vi "get_data.vi"(11 "JSON":variant) -> (0 "Standards [%]":map{string, i32}(c390), 1 "Indexes":map{string, variant}(c390), 3 "Conditions":map{string, i32}(c390), 5 "Timestamps":map{string, string}(c390))   [LabVIEW 2019]
uses:
  <vilib>/LVH/i3 JSON/JSON Parsing/Get Object Parameter Files/Get Object Parameter - Array.vi
  <vilib>/LVH/i3 JSON/JSON Parsing/Get Array Value at Index Files/Get Array Value at Index - Object.vi
  <vilib>/LVH/i3 JSON/JSON Parsing/Get Object Parameter Files/Get Object Parameter - Numeric.vi
  <vilib>/LVH/i3 JSON/JSON Parsing/Get Object Parameter Files/Get Object Parameter - String.vi
  <vilib>/LVH/i3 JSON/JSON Parsing/Get Object Parameter Files/Get Object Parameter - Object.vi
  <vilib>/LVH/i3 JSON/i3-json.lvlib
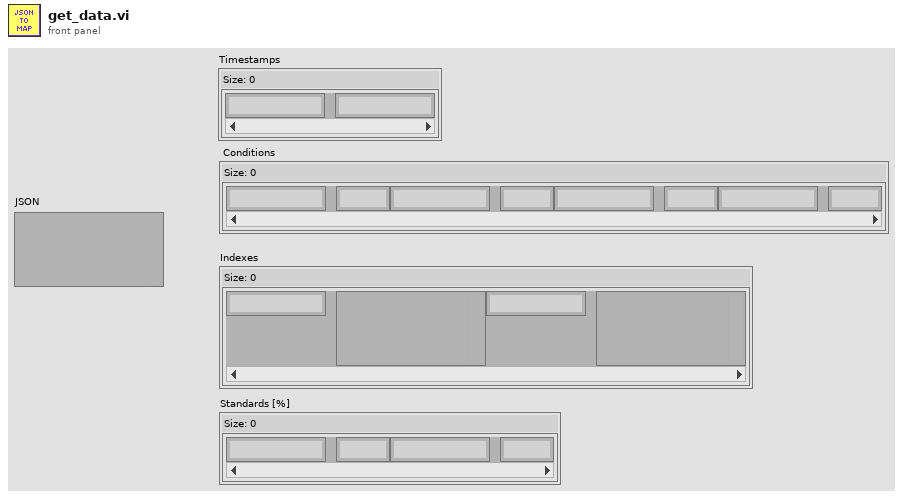
[diagram p1: front panel]
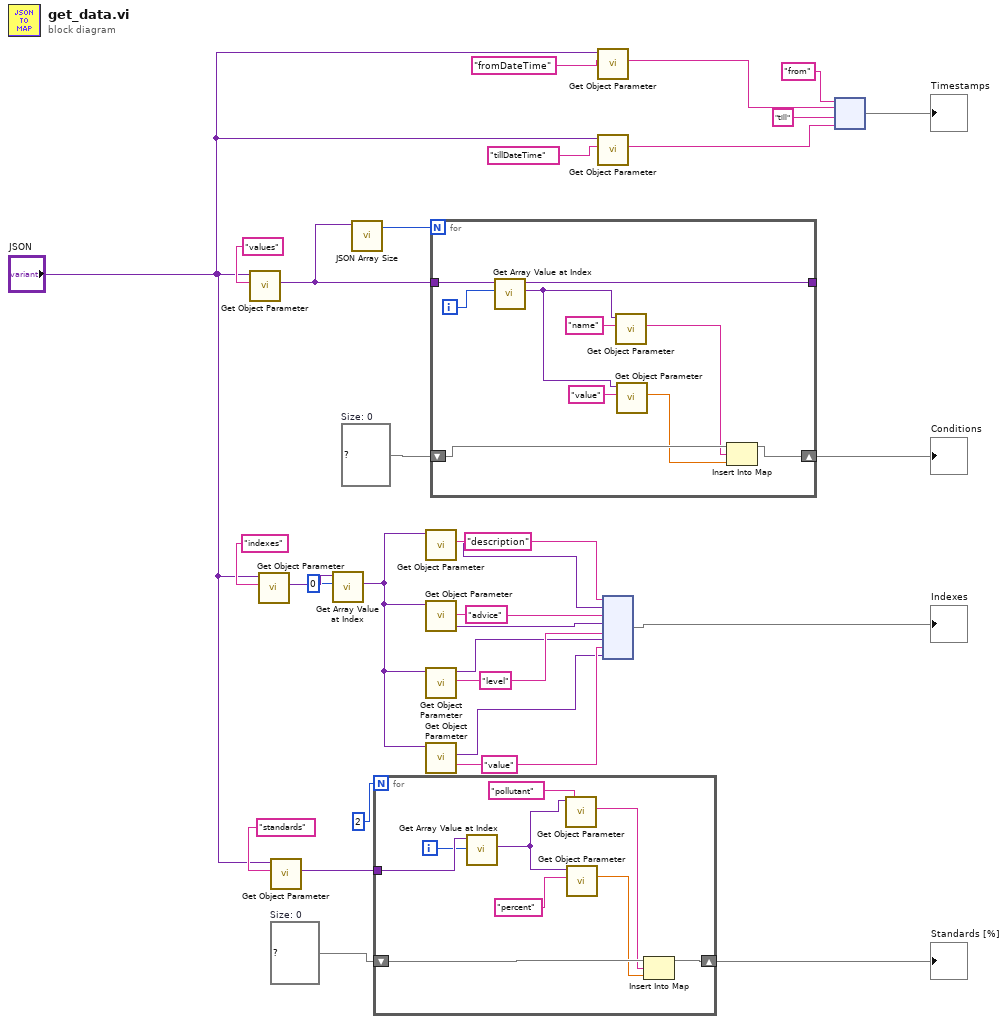
[diagram p0: block diagram]
diagram:
  w10 = map{string, i32} {}  # Size: 0
  w15 = "value" ("Parameter Name")
  w18 = "level" ("Parameter Name")
  w20 = "advice" ("Parameter Name")
  w22 = "description" ("Parameter Name")
  w28 = map{string, i32} {}  # Size: 0
  n1 = call-poly <vilib>:"Get Object Parameter.vi"("Parameter Name"="values", "JSON Tree In (JSON Object)"="JSON") -> ("JSON Array"=w29:variant)  [unwired: 6 in, 3 out]
  n2 = call-poly <vilib>:"Get Object Parameter.vi"("Parameter Name"="indexes", "JSON Tree In (JSON Object)"="JSON") -> ("JSON Array"=w26:variant)  [unwired: 6 in, 3 out]
  n3 = call-poly <vilib>:"Get Object Parameter.vi"("Parameter Name"="standards", "JSON Tree In (JSON Object)"="JSON") -> ("JSON Array"=w12:variant)  [unwired: 6 in, 3 out]
  n4 = call-poly <vilib>:"Get Array Value at Index.vi"("Index"=0, "JSON Tree In (JSON Array)"=w26) -> ("JSON Object"=w23:variant)  [unwired: 6 in, 3 out]
  n5 = call <vilib>:"JSON Array Size.vi"("JSON Tree In (JSON Array)"=w29) -> ("Array Size"=w30:i32)  [unwired: 8 in, 2 out]
  n6 = for {
    N: 2 -> [_]
    tunnel: w12 -> [w40]
    shift-right: [w37] -> w9
    shift-left: w10 -> [w38]
    i -> [w39]
    n7 = call-poly <vilib>:"Get Array Value at Index.vi"("Index"=w39, "JSON Tree In (JSON Array)"=w40) -> ("JSON Object"=w32:variant)  [unwired: 6 in, 3 out]
    n8 = call-poly <vilib>:"Get Object Parameter.vi"("Parameter Name"="pollutant", "JSON Tree In (JSON Object)"=w32) -> ("String Value"=w33:string)  [unwired: 6 in, 3 out]
    n9 = call-poly <vilib>:"Get Object Parameter.vi"("Parameter Name"="percent", "JSON Tree In (JSON Object)"=w32) -> ("Double Value"=w34:dbl)  [unwired: 6 in, 3 out]
    n10 = Insert Into Map(map in=w38, key=w33, value=w34) -> (map out=w37:map{string, i32})  [unwired: 2 out]
  }
  "Standards [%]" <- w9
  n11 = call-poly <vilib>:"Get Object Parameter.vi"("Parameter Name"=w22, "JSON Tree In (JSON Object)"=w23) -> ("JSON Object"=w21:variant)  [unwired: 6 in, 3 out]
  n12 = call-poly <vilib>:"Get Object Parameter.vi"("Parameter Name"=w20, "JSON Tree In (JSON Object)"=w23) -> ("JSON Object"=w17:variant)  [unwired: 6 in, 3 out]
  n13 = call-poly <vilib>:"Get Object Parameter.vi"("Parameter Name"=w18, "JSON Tree In (JSON Object)"=w23) -> ("JSON Tree Out Passthrough"=w16:variant)  [unwired: 6 in, 3 out]
  n14 = call-poly <vilib>:"Get Object Parameter.vi"("Parameter Name"=w15, "JSON Tree In (JSON Object)"=w23) -> ("JSON Object"=w14:variant)  [unwired: 6 in, 3 out]
  n15 = for {
    N: w30 -> [_]
    tunnel: w29 -> [w50]
    tunnel: [w48] -> _
    shift-right: [w43] -> w24
    shift-left: w28 -> [w44]
    i -> [w49]
    n16 = call-poly <vilib>:"Get Array Value at Index.vi"("Index"=w49, "JSON Tree In (JSON Array)"=w50) -> ("JSON Object"=w45:variant, "JSON Tree Out Passthrough"=w48:variant)  [unwired: 6 in, 2 out]
    n17 = call-poly <vilib>:"Get Object Parameter.vi"("Parameter Name"="name", "JSON Tree In (JSON Object)"=w45) -> ("String Value"=w42:string)  [unwired: 6 in, 3 out]
    n18 = call-poly <vilib>:"Get Object Parameter.vi"("Parameter Name"="value", "JSON Tree In (JSON Object)"=w45) -> ("Double Value"=w41:dbl)  [unwired: 6 in, 3 out]
    n19 = Insert Into Map(map in=w44, key=w42, value=w41) -> (map out=w43:map{string, i32})  [unwired: 2 out]
  }
  "Conditions" <- w24
  n20 = call-poly <vilib>:"Get Object Parameter.vi"("Parameter Name"="fromDateTime", "JSON Tree In (JSON Object)"="JSON") -> ("String Value"=w4:string)  [unwired: 6 in, 3 out]
  n21 = call-poly <vilib>:"Get Object Parameter.vi"("Parameter Name"="tillDateTime", "JSON Tree In (JSON Object)"="JSON") -> ("String Value"=w3:string)  [unwired: 6 in, 3 out]
  n22 = node(w22, w21, w20, w17, w18, w16, w15, w14) -> (→"Indexes":map{string, variant})
  n23 = node("from" ("key"), w4, "till" ("key"), w3) -> (→"Timestamps":map{string, string})
